vi "Main.vi"() -> ()   [LabVIEW 2011]
uses:
  ReadingsCtrl.ctl
panel:
  in  "Set 2":bool
  in  "!st Set":bool
  out "Interlock 2":bool
  out "FLW_IL 2":bool
  out "COND_IL 2":bool
  out "KLXON_IL 2":bool
  out "TMP_IL 2":bool
  out "Remote ON 2":bool
  out "HMIRST 2":bool
  in  "Read 2":bool
  in  "Read":bool
  out "Readings 2":T1
  out "Readings":T1
  in  "dec":bool
  in  "inc":bool
  out "Message":string
  in  "HMI Reset":bool
  out "Enable RESET after error":bool
  out "Mag ON OFF Status":bool
  in  "Remote Turn ONOFF":bool
  out "HMIRST":bool
  out "Interlock":bool
  out "Remote ON":bool
  out "TMP_IL":bool
  out "KLXON_IL":bool
  out "COND_IL":bool
  out "FLW_IL":bool
  in  "error in (no error)":errorcluster
  in  "HMI PWR":u16
  in  "stop":bool
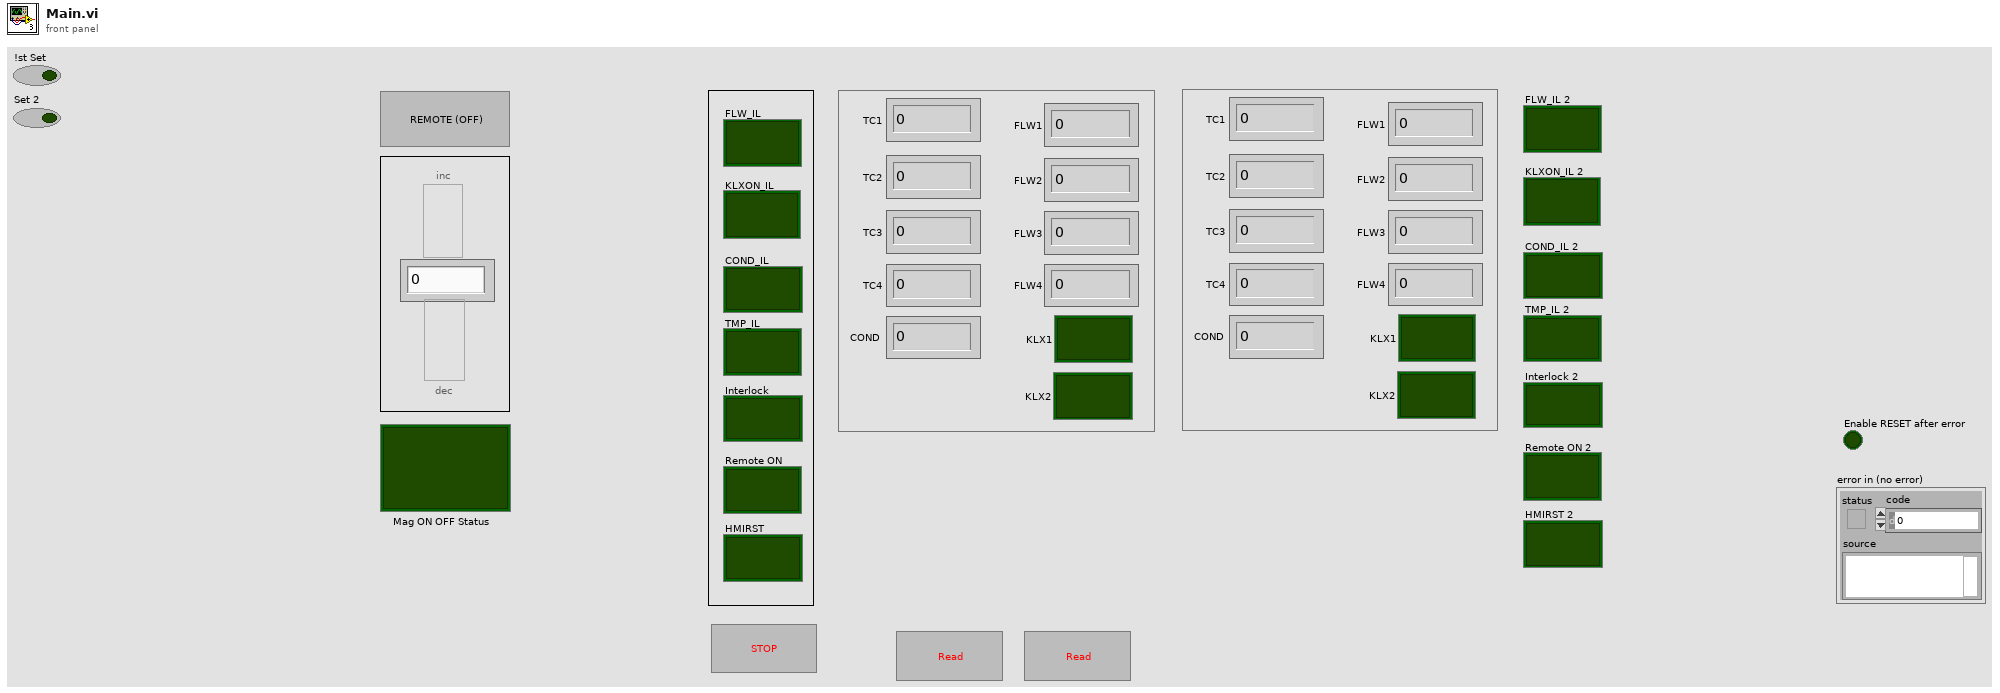
[diagram p1: front panel]
types:
  T1 = typedef "ReadingsCtrl.ctl" = cluster{"TC1":u16, "TC2":u16, "TC3":u16, "TC4":u16, "FLW1":u16, "FLW2":u16, "FLW3":u16, "FLW4":u16, "COND":u16, "KLX1":bool, "KLX2":bool}
  T2 = cluster{"Enable Reset HMI":bool, "Power Val":u16}
  T3 = enum8{"Enabled", "Disabled", "Disabled and Grayed Out"}
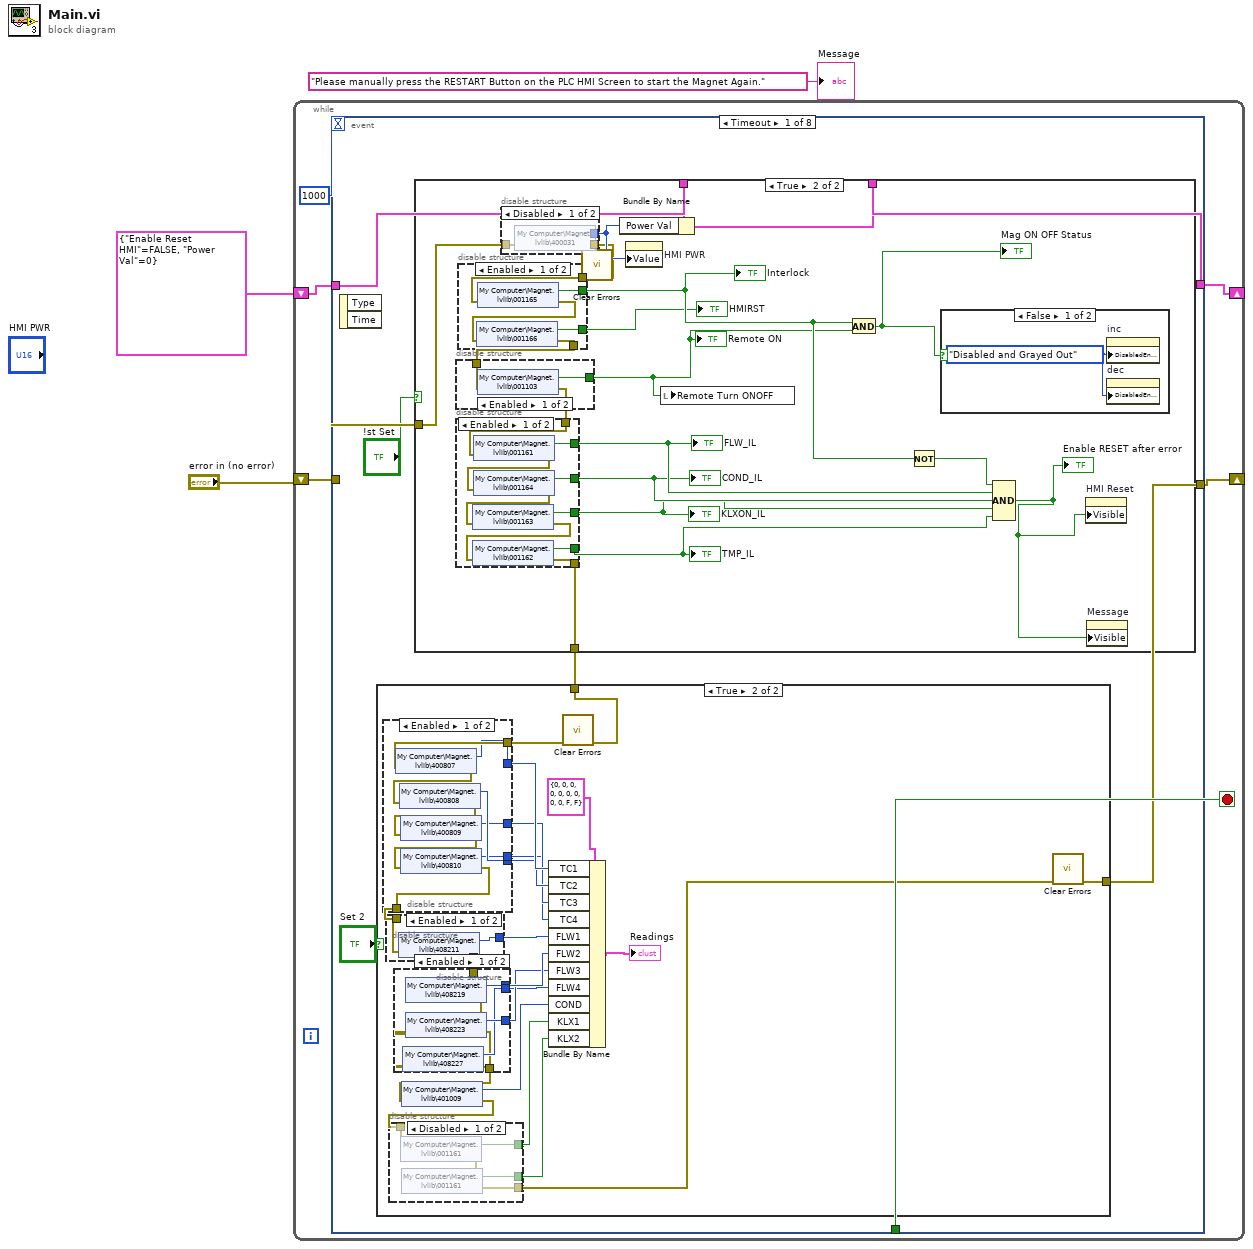
[diagram p0: block diagram]
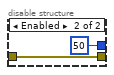
[diagram p11: hidden frame]
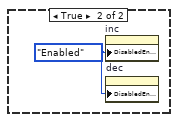
[diagram p12: hidden frame]
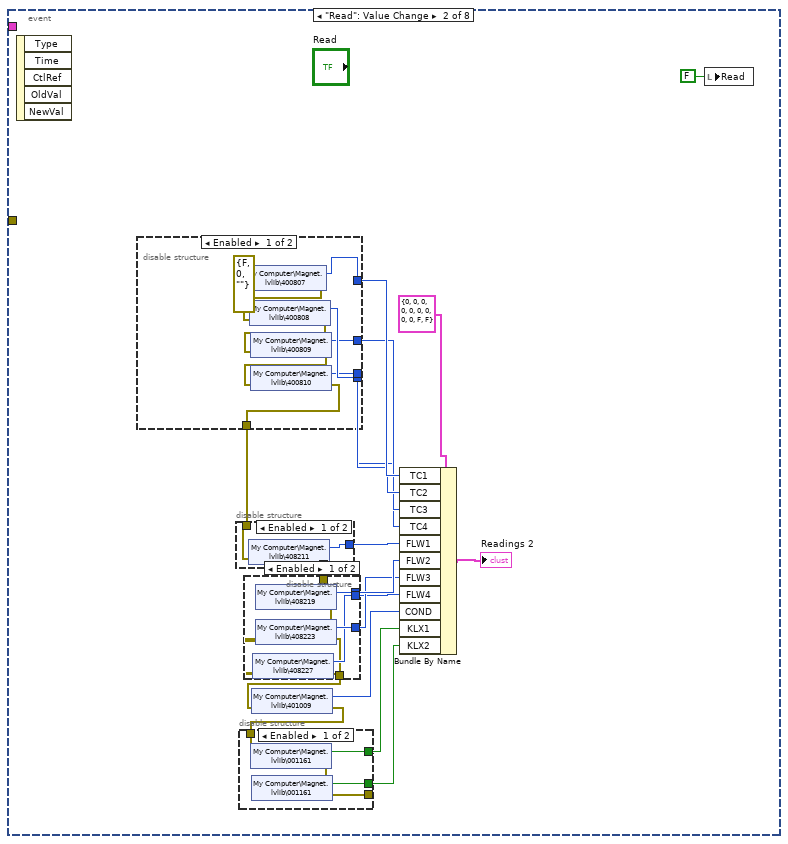
[diagram p13: hidden frame]
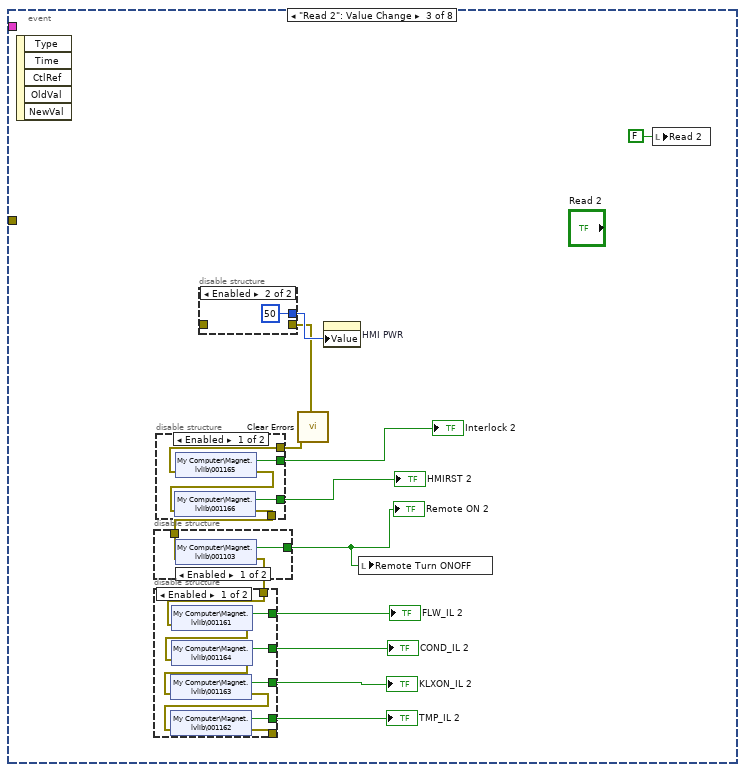
[diagram p18: hidden frame]
diagram:
  n1 = while {
    shift-right: [w7] -> _
    shift-left: "error in (no error)" -> [w8]
    shift-right: [w4] -> _
    shift-left: T2 {"Enable Reset HMI"=FALSE, "Power Val"=0} -> [w5]
    stop <- w9 stop-if-true
    n2 = event shown="[0] Timeout" {
      selector: _ -> [_ _ _ _ _ _ _ _]
      dyn-events: _ -> [_ _ _ _ _ _ _ _]
      timeout: 1000 -> [_ _ _ _ _ _ _ _]
      tunnel: [_ _ _ _ _ _ TRUE _] -> w9
      tunnel: [w13 _ _ w192 w206 w216 w221 w225] -> w7
      tunnel: w8 -> [w14 _ _ w191 w205 w215 w221 w227]
      tunnel: w5 -> [w16 _ _ w193 w207 _ _ _]
      tunnel: [w15 _ _ w193 w207 _ _ _] -> w4
      event Timeout {
        n3 = event-data() -> ()  [unwired: 1 in, 2 out]
        n4 = case shown="True" "!st Set" {
          tunnel: w16 -> [w65 w74]
          tunnel: [w65 w73] -> w15
          tunnel: w14 -> [w64 w71]
          tunnel: [w64 w68] -> w12
          frame False {
          }
          frame True {
            n5 = disable-structure shown="Disabled" {
              disable-tunnel: [w106 u16 50] -> w72
              disable-tunnel: w71 -> [w105 w108]
              disable-tunnel: [w104 w108] -> w69
              frame Disabled {
                n6 = shared-variable "My Computer\\Magnet.lvlib\\400031"(error in=w105) -> (w106:u16, error out=w104:errorcluster)
              }
              frame Enabled {
              }
            }
            n7 = call <vilib>:"Clear Errors.vi"("error in (no error)"=w69) -> ("error out"=w66:errorcluster)  [unwired: 6 in]
            n8 = disable-structure shown="Enabled" {
              disable-tunnel: [w102 _] -> w84
              disable-tunnel: [w101 _] -> w83
              disable-tunnel: [w99 w103] -> w70
              disable-tunnel: w66 -> [w98 w103]
              frame Enabled {
                n9 = shared-variable "My Computer\\Magnet.lvlib\\001165"(error in=w98) -> (w102:bool, error out=w100:errorcluster)
                n10 = shared-variable "My Computer\\Magnet.lvlib\\001166"(error in=w100) -> (w101:bool, error out=w99:errorcluster)
              }
              frame Disabled {
              }
            }
            "Interlock" <- w84
            "HMIRST" <- w83
            n11 = disable-structure shown="Enabled" {
              disable-tunnel: [w87 _] -> w75
              disable-tunnel: w70 -> [w86 _]
              disable-tunnel: [w85 _] -> w67
              frame Enabled {
                n12 = shared-variable "My Computer\\Magnet.lvlib\\001103"(error in=w86) -> (w87:bool, error out=w85:errorcluster)
              }
              frame Disabled {
              }
            }
            "Remote ON" <- w75
            n13 = disable-structure shown="Enabled" {
              disable-tunnel: [w96 _] -> w81
              disable-tunnel: [w95 _] -> w80
              disable-tunnel: [w94 _] -> w79
              disable-tunnel: [w93 _] -> w78
              disable-tunnel: [w92 w97] -> w68
              disable-tunnel: w67 -> [w91 w97]
              frame Enabled {
                n14 = shared-variable "My Computer\\Magnet.lvlib\\001161"(error in=w91) -> (w96:bool, error out=w90:errorcluster)
                n15 = shared-variable "My Computer\\Magnet.lvlib\\001164"(error in=w90) -> (w95:bool, error out=w89:errorcluster)
                n16 = shared-variable "My Computer\\Magnet.lvlib\\001163"(error in=w89) -> (w94:bool, error out=w88:errorcluster)
                n17 = shared-variable "My Computer\\Magnet.lvlib\\001162"(error in=w88) -> (w93:bool, error out=w92:errorcluster)
              }
              frame Disabled {
              }
            }
            "FLW_IL" <- w81
            "COND_IL" <- w80
            "KLXON_IL" <- w79
            "TMP_IL" <- w78
            n18 = Bundle By Name(cluster=w74, "Power Val"=w72) -> (w73:T2)
            n19 = property on="HMI PWR" class="DigNum (strict)"("Value"=w72) -> ()  [unwired: 2 in, 2 out]
            n20 = local write "Remote Turn ONOFF"(w75) -> ()
            n21 = And(x=w84, y=w75) -> (x .and. y?=w76:bool)
            "Mag ON OFF Status" <- w76
            n22 = Not(x=w84) -> (.not. x?=w82:bool)
            n23 = case shown="False" w76 {
              frame False {
                w109 = T3."Disabled and Grayed Out" ("Disabled")
                n24 = property on="inc" class="Bool (strict)"("DisabledEnum"=w109) -> ()  [unwired: 2 in, 2 out]
                n25 = property on="dec" class="Bool (strict)"("DisabledEnum"=w109) -> ()  [unwired: 2 in, 2 out]
              }
              frame True {
                w110 = T3."Enabled" ("Disabled")
                n26 = property on="inc" class="Bool (strict)"("DisabledEnum"=w110) -> ()  [unwired: 2 in, 2 out]
                n27 = property on="dec" class="Bool (strict)"("DisabledEnum"=w110) -> ()  [unwired: 2 in, 2 out]
              }
            }
            n28 = Compound Arithmetic op=AND(w82, w81, w80, w79, w78) -> (w77:bool)
            "Enable RESET after error" <- w77
            n29 = property on="HMI Reset" class="Bool (strict)"("Visible"=w77) -> ()  [unwired: 2 in, 2 out]
            n30 = property on="Message" class="Str"("Visible"=w77) -> ()  [unwired: 2 in, 2 out]
          }
        }
        n31 = case shown="True" "Set 2" {
          tunnel: [w17 w38] -> w13
          tunnel: w12 -> [w17 w37]
          frame False {
          }
          frame True {
            n32 = call <vilib>:"Clear Errors.vi"("error in (no error)"=w37) -> ("error out"=w18:errorcluster)  [unwired: 6 in]
            n33 = disable-structure shown="Enabled" {
              disable-tunnel: w18 -> [w63 _]
              disable-tunnel: [w62 _] -> w33
              disable-tunnel: [w61 _] -> w31
              disable-tunnel: [w60 _] -> w30
              disable-tunnel: [w59 _] -> w29
              disable-tunnel: [w55 _] -> w20
              frame Enabled {
                n34 = shared-variable "My Computer\\Magnet.lvlib\\400807"(error in=w63) -> (w62:u16, error out=w58:errorcluster)
                n35 = shared-variable "My Computer\\Magnet.lvlib\\400808"(error in=w58) -> (w61:u16, error out=w56:errorcluster)
                n36 = shared-variable "My Computer\\Magnet.lvlib\\400809"(error in=w56) -> (w60:u16, error out=w57:errorcluster)
                n37 = shared-variable "My Computer\\Magnet.lvlib\\400810"(error in=w57) -> (w59:u16, error out=w55:errorcluster)
              }
              frame Disabled {
              }
            }
            n38 = disable-structure shown="Enabled" {
              disable-tunnel: [w54 _] -> w28
              disable-tunnel: [w53 _] -> w23
              disable-tunnel: w20 -> [w52 _]
              frame Enabled {
                n39 = shared-variable "My Computer\\Magnet.lvlib\\408211"(error in=w52) -> (w54:u16, error out=w53:errorcluster)
              }
              frame Disabled {
              }
            }
            n40 = disable-structure shown="Enabled" {
              disable-tunnel: [w51 _] -> w27
              disable-tunnel: [w50 _] -> w26
              disable-tunnel: [w49 _] -> w25
              disable-tunnel: w23 -> [w48 _]
              disable-tunnel: [w45 _] -> w22
              frame Enabled {
                n41 = shared-variable "My Computer\\Magnet.lvlib\\408219"(error in=w48) -> (w51:u16, error out=w47:errorcluster)
                n42 = shared-variable "My Computer\\Magnet.lvlib\\408223"(error in=w47) -> (w50:u16, error out=w46:errorcluster)
                n43 = shared-variable "My Computer\\Magnet.lvlib\\408227"(error in=w46) -> (w49:u16, error out=w45:errorcluster)
              }
              frame Disabled {
              }
            }
            n44 = shared-variable "My Computer\\Magnet.lvlib\\401009"(error in=w22) -> (w24:u16, error out=w21:errorcluster)
            n45 = disable-structure shown="Disabled" {
              disable-tunnel: [w43 w44] -> w19
              disable-tunnel: [w42 _] -> w36
              disable-tunnel: [w41 _] -> w35
              disable-tunnel: w21 -> [w39 w44]
              frame Disabled {
                n46 = shared-variable "My Computer\\Magnet.lvlib\\001161"(error in=w39) -> (w41:bool, error out=w40:errorcluster)
                n47 = shared-variable "My Computer\\Magnet.lvlib\\001161"(error in=w40) -> (w42:bool, error out=w43:errorcluster)
              }
              frame Enabled {
              }
            }
            n48 = Bundle By Name(cluster=T1 {"TC1"=0, "TC2"=0, "TC3"=0, "TC4"=0, "FLW1"=0, "FLW2"=0, "FLW3"=0, "FLW4"=0, "COND"=0, "KLX1"=FALSE, "KLX2"=FALSE} ("Readings"), "TC1"=w33, "TC2"=w31, "TC3"=w30, "TC4"=w29, "FLW1"=w28, "FLW2"=w27, "FLW3"=w26, "FLW4"=w25, "COND"=w24, "KLX1"=w35, "KLX2"=w36) -> (→"Readings":T1)
            n49 = call <vilib>:"Clear Errors.vi"("error in (no error)"=w19) -> ("error out"=w38:errorcluster)  [unwired: 6 in]
          }
        }
      }
      event "Read": Value Change {
        n50 = event-data() -> ()  [unwired: 1 in, 5 out]
        n51 = disable-structure shown="Enabled" {
          disable-tunnel: [w153 _] -> w125
          disable-tunnel: [w152 _] -> w123
          disable-tunnel: [w151 _] -> w122
          disable-tunnel: [w150 _] -> w121
          disable-tunnel: [w146 _] -> w112
          frame Enabled {
            n52 = shared-variable "My Computer\\Magnet.lvlib\\400807"(error in=errorcluster {"status"=FALSE, "code"=0, "source"=""} ("error in (no error)")) -> (w153:u16, error out=w149:errorcluster)
            n53 = shared-variable "My Computer\\Magnet.lvlib\\400808"(error in=w149) -> (w152:u16, error out=w147:errorcluster)
            n54 = shared-variable "My Computer\\Magnet.lvlib\\400809"(error in=w147) -> (w151:u16, error out=w148:errorcluster)
            n55 = shared-variable "My Computer\\Magnet.lvlib\\400810"(error in=w148) -> (w150:u16, error out=w146:errorcluster)
          }
          frame Disabled {
          }
        }
        n56 = disable-structure shown="Enabled" {
          disable-tunnel: [w144 _] -> w120
          disable-tunnel: [w143 _] -> w115
          disable-tunnel: w112 -> [w142 _]
          frame Enabled {
            n57 = shared-variable "My Computer\\Magnet.lvlib\\408211"(error in=w142) -> (w144:u16, error out=w143:errorcluster)
          }
          frame Disabled {
          }
        }
        n58 = disable-structure shown="Enabled" {
          disable-tunnel: [w141 _] -> w119
          disable-tunnel: [w140 _] -> w118
          disable-tunnel: [w139 _] -> w117
          disable-tunnel: w115 -> [w138 _]
          disable-tunnel: [w135 _] -> w114
          frame Enabled {
            n59 = shared-variable "My Computer\\Magnet.lvlib\\408219"(error in=w138) -> (w141:u16, error out=w137:errorcluster)
            n60 = shared-variable "My Computer\\Magnet.lvlib\\408223"(error in=w137) -> (w140:u16, error out=w136:errorcluster)
            n61 = shared-variable "My Computer\\Magnet.lvlib\\408227"(error in=w136) -> (w139:u16, error out=w135:errorcluster)
          }
          frame Disabled {
          }
        }
        n62 = shared-variable "My Computer\\Magnet.lvlib\\401009"(error in=w114) -> (w116:u16, error out=w113:errorcluster)
        n63 = disable-structure shown="Enabled" {
          disable-tunnel: [w133 w134] -> _
          disable-tunnel: [w132 _] -> w128
          disable-tunnel: [w131 _] -> w127
          disable-tunnel: w113 -> [w129 w134]
          frame Enabled {
            n64 = shared-variable "My Computer\\Magnet.lvlib\\001161"(error in=w129) -> (w131:bool, error out=w130:errorcluster)
            n65 = shared-variable "My Computer\\Magnet.lvlib\\001161"(error in=w130) -> (w132:bool, error out=w133:errorcluster)
          }
          frame Disabled {
          }
        }
        n66 = Bundle By Name(cluster=T1 {"TC1"=0, "TC2"=0, "TC3"=0, "TC4"=0, "FLW1"=0, "FLW2"=0, "FLW3"=0, "FLW4"=0, "COND"=0, "KLX1"=FALSE, "KLX2"=FALSE} ("Readings"), "TC1"=w125, "TC2"=w123, "TC3"=w122, "TC4"=w121, "FLW1"=w120, "FLW2"=w119, "FLW3"=w118, "FLW4"=w117, "COND"=w116, "KLX1"=w127, "KLX2"=w128) -> (→"Readings 2":T1)
        n67 = local write "Read"(FALSE ("Read")) -> ()
      }
      event "Read 2": Value Change {
        n68 = event-data() -> ()  [unwired: 1 in, 5 out]
        n69 = disable-structure shown="Enabled" {
          disable-tunnel: [w188 u16 50] -> w159
          disable-tunnel: _ -> [w187 _]
          disable-tunnel: [w186 _] -> w157
          frame Disabled {
            n70 = shared-variable "My Computer\\Magnet.lvlib\\400031"(error in=w187) -> (w188:u16, error out=w186:errorcluster)
          }
          frame Enabled {
          }
        }
        n71 = call <vilib>:"Clear Errors.vi"("error in (no error)"=w157) -> ("error out"=w155:errorcluster)  [unwired: 6 in]
        n72 = disable-structure shown="Enabled" {
          disable-tunnel: [w184 _] -> w166
          disable-tunnel: [w183 _] -> w165
          disable-tunnel: [w181 w185] -> w158
          disable-tunnel: w155 -> [w180 w185]
          frame Enabled {
            n73 = shared-variable "My Computer\\Magnet.lvlib\\001165"(error in=w180) -> (w184:bool, error out=w182:errorcluster)
            n74 = shared-variable "My Computer\\Magnet.lvlib\\001166"(error in=w182) -> (w183:bool, error out=w181:errorcluster)
          }
          frame Disabled {
          }
        }
        "Interlock 2" <- w166
        "HMIRST 2" <- w165
        n75 = disable-structure shown="Enabled" {
          disable-tunnel: [w169 _] -> w160
          disable-tunnel: w158 -> [w168 _]
          disable-tunnel: [w167 _] -> w156
          frame Enabled {
            n76 = shared-variable "My Computer\\Magnet.lvlib\\001103"(error in=w168) -> (w169:bool, error out=w167:errorcluster)
          }
          frame Disabled {
          }
        }
        "Remote ON 2" <- w160
        n77 = disable-structure shown="Enabled" {
          disable-tunnel: [w178 _] -> w164
          disable-tunnel: [w177 _] -> w163
          disable-tunnel: [w176 _] -> w162
          disable-tunnel: [w175 _] -> w161
          disable-tunnel: [w174 w179] -> _
          disable-tunnel: w156 -> [w173 w179]
          frame Enabled {
            n78 = shared-variable "My Computer\\Magnet.lvlib\\001161"(error in=w173) -> (w178:bool, error out=w172:errorcluster)
            n79 = shared-variable "My Computer\\Magnet.lvlib\\001164"(error in=w172) -> (w177:bool, error out=w171:errorcluster)
            n80 = shared-variable "My Computer\\Magnet.lvlib\\001163"(error in=w171) -> (w176:bool, error out=w170:errorcluster)
            n81 = shared-variable "My Computer\\Magnet.lvlib\\001162"(error in=w170) -> (w175:bool, error out=w174:errorcluster)
          }
          frame Disabled {
          }
        }
        "FLW_IL 2" <- w164
        "COND_IL 2" <- w163
        "KLXON_IL 2" <- w162
        "TMP_IL 2" <- w161
        n82 = property on="HMI PWR" class="DigNum (strict)"("Value"=w159) -> ()  [unwired: 2 in, 2 out]
        n83 = local write "Remote Turn ONOFF"(w160) -> ()
        n84 = local write "Read 2"(FALSE ("Read 2")) -> ()
      }
      event "inc": Value Change {
        n85 = event-data() -> ()  [unwired: 1 in, 5 out]
        n86 = Unbundle By Name(w193) -> ("Power Val"=w194:u16)
        n87 = Greater?(x=w194, y=u16 800) -> (0:w195:bool)
        n88 = case shown="False" w195 {
          tunnel: w194 -> [w201 _]
          tunnel: [w197 w202] -> w192
          tunnel: w191 -> [_ w202]
          frame False {
            n89 = Add(x=w201, y=u16 50) -> (x+y=w199:u16)
            n90 = shared-variable "My Computer\\Magnet.lvlib\\400004"(w199) -> (error out=w198:errorcluster)  [unwired: 1 in]
            n91 = property on="HMI PWR" class="DigNum (strict)"("Value"=w199) -> ()  [unwired: 2 in, 2 out]
            n92 = call <vilib>:"Clear Errors.vi"("error in (no error)"=w198) -> ("error out"=w197:errorcluster)  [unwired: 6 in]
          }
          frame True {
          }
        }
        n93 = local write "inc"(FALSE ("inc")) -> ()
      }
      event "dec": Value Change {
        n94 = event-data() -> ()  [unwired: 1 in, 5 out]
        n95 = Unbundle By Name(w207) -> ("Power Val"=w204:u16)
        n96 = Less Or Equal To 0?(x=w204) -> (x <= 0?=w208:bool)
        n97 = case shown="False" w208 {
          tunnel: w204 -> [w213 _]
          tunnel: [w209 w214] -> w206
          tunnel: w205 -> [_ w214]
          frame False {
            n98 = Subtract(x=w213, y=u16 50) -> (x-y=w211:u16)
            n99 = shared-variable "My Computer\\Magnet.lvlib\\400004"(w211) -> (error out=w210:errorcluster)  [unwired: 1 in]
            n100 = property on="HMI PWR" class="DigNum (strict)"("Value"=w211) -> ()  [unwired: 2 in, 2 out]
            n101 = call <vilib>:"Clear Errors.vi"("error in (no error)"=w210) -> ("error out"=w209:errorcluster)  [unwired: 6 in]
          }
          frame True {
            # "Do not set value below zero"
          }
        }
        n102 = local write "dec"(FALSE ("dec")) -> ()
      }
      event "HMI Reset": Value Change {
        n103 = event-data() -> ()  [unwired: 1 in, 5 out]
        n104 = flat-sequence {
          tunnel: [w218] -> w216
          tunnel: w215 -> [w217]
          frame #0 {
            n105 = shared-variable "My Computer\\Magnet.lvlib\\001166"(TRUE ("400006.2"), error in=w217) -> (error out=w219:errorcluster)
            n106 = call <vilib>:"Clear Errors.vi"("error in (no error)"=w219) -> ("error out"=w218:errorcluster)  [unwired: 6 in]
          }
          frame #1 {
          }
          frame #2 {
          }
        }
      }
      event "stop": Value Change {
        n107 = event-data() -> ()  [unwired: 1 in, 5 out]
        n108 = local write "stop"(FALSE ("stop")) -> ()
      }
      event "Remote Turn ONOFF": Value Change {
        n109 = event-data() -> ("NewVal"=w224:bool)  [unwired: 1 in, 4 out]
        n110 = shared-variable "My Computer\\Magnet.lvlib\\001103"(w224, error in=w227) -> (error out=w226:errorcluster)
        n111 = call <vilib>:"Clear Errors.vi"("error in (no error)"=w226) -> ("error out"=w225:errorcluster)  [unwired: 6 in]
      }
    }
  }
  "Message" <- "Please manually press the RESTART Button on the PLC HMI Screen to start the Magnet Again." ("String")
